vi "Get End Tag.vi"(8 "error in (no error)":errorcluster, 10 "Name":string, 11 "Element in":refnum<class "Element.lvclass">) -> (0 "error out":errorcluster, 2 "End Tag":string, 3 "Element out":refnum<class "Element.lvclass">)   [LabVIEW 2026, in "VILab.lvlib" / "Element.lvclass"]
uses:
  Element.lvclass
  Data Item/Data Item.lvclass
  Element.lvclass/Element.ctl
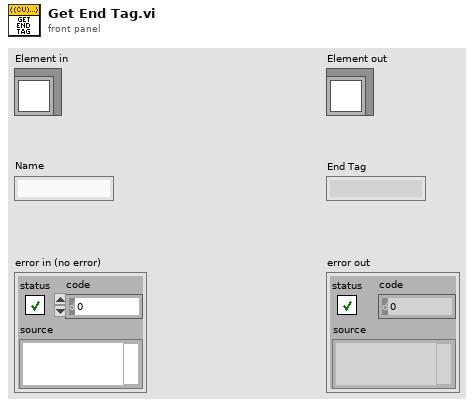
[diagram p1: front panel]
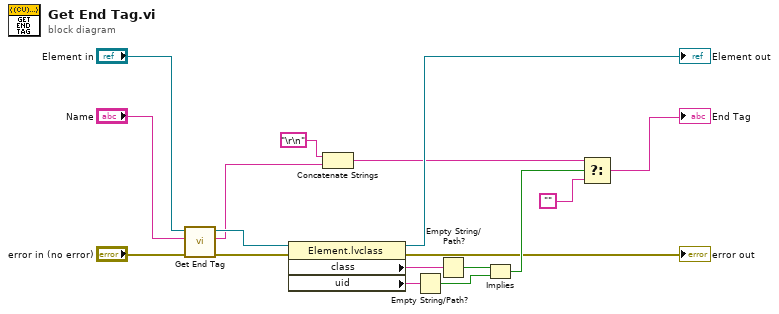
[diagram p0: block diagram]
diagram:
  n1 = call-parent "Get End Tag.vi"("error in (no error)"="error in (no error)", "Name"="Name", "Data Item in"="Element in") -> ("error out"=w9:errorcluster, "End Tag"=w7:string, "Data Item out"=w10:refnum<class "Element.lvclass">)  [unwired: 6 in]
  n2 = property class="Element.lvclass"(reference=w10, error in=w9) -> (reference out=→"Element out":refnum<class "Element.lvclass">, error out=→"error out":errorcluster, "class"=w16:string, "uid"=w15:string)
  n3 = Concatenate Strings("\r\n", w7) -> (w3:string)
  n4 = Empty String/Path?(string/path=w15) -> (empty?=w13:bool)
  n5 = Empty String/Path?(string/path=w16) -> (empty?=w14:bool)
  n6 = Implies(1:w13, 2:w14) -> (0:w5:bool)
  n7 = Select(t=w3, s=w5, f="") -> (s? t:f=→"End Tag":string)
